vi "N Point Running Average.vi"(1 "n":i8, 2 "Input":dbl) -> (0 "Output":dbl)   [LabVIEW 2015]
uses:
  <vilib>/Analysis/baseanly.llb/Mean (DBL).vi
  <vilib>/Analysis/NI_AALBase.lvlib
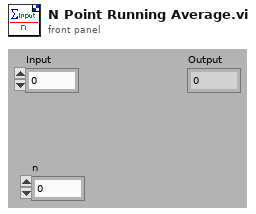
[diagram p1: front panel]
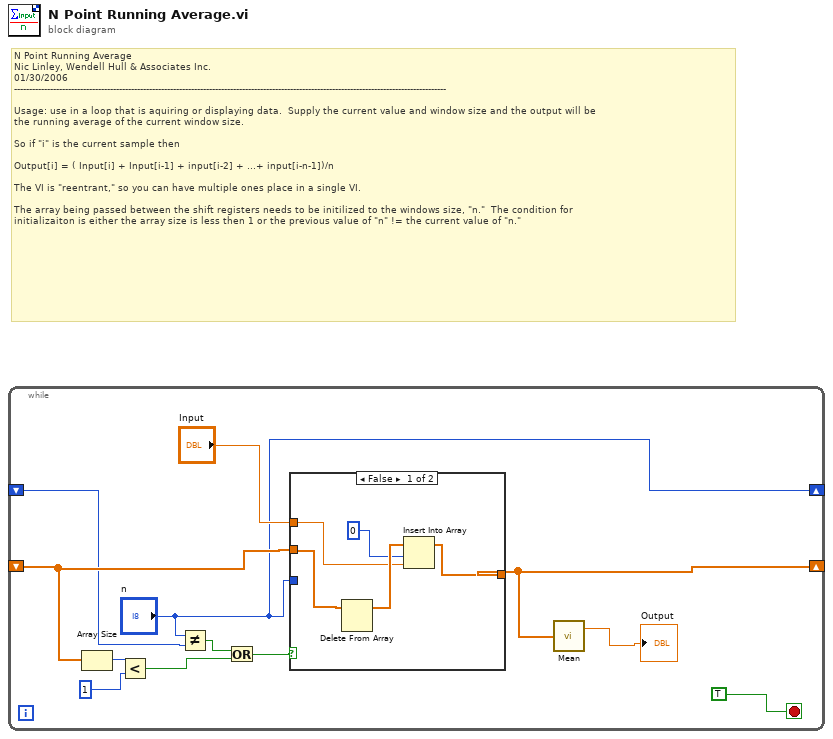
[diagram p0: block diagram]
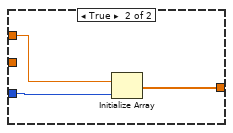
[diagram p2: hidden frame]
diagram:
  # "N Point Running Average \nNic Linley, Wendell Hull & Associates Inc.\n01/30/2006\n------------------------------------------------------------------------------------------------------------------------------------------------\n\nUsage: use in a loop that is aquiring or displaying data.  Supply the current value and window size and the output will be\nthe running average of the current window size.\n\nSo if \"i\" is the current sample then\n\nOutput[i] = ( Input[i] + Input[i-1] + input[i-2] + ...+ input[i-n-1])/n\n\nThe VI is \"reentrant,\" so you can have multiple ones place in a single VI.\n\nThe array being passed between the shift registers needs to be initilized to the windows size, \"n.\"  The condition for\ninitializaiton is either the array size is less then 1 or the previous value of \"n\" != the current value of \"n.\""
  n1 = while {
    shift-right: [w8] -> _
    shift-left: _ -> [w9]
    shift-right: ["n"] -> _
    shift-left: _ -> [w3]
    stop <- TRUE stop-if-true
    n2 = Array Size(array=w9) -> (size(s)=w11:i32)
    n3 = Less?(x=w11, y=1) -> (x < y?=w1:bool)
    n4 = Not Equal?(x="n", y=w3) -> (x != y?=w2:bool)
    n5 = Or(x=w2, y=w1) -> (x .or. y?=w5:bool)
    n6 = case shown="False" w5 {
      tunnel: "n" -> [_ w20]
      tunnel: "Input" -> [w15 w19]
      tunnel: [w14 w18] -> w8
      tunnel: w9 -> [w17 _]
      frame False {
        n7 = Delete From Array "Delete From Array"(array=w17) -> (array with subset deleted=w16:dbl[])  [unwired: 2 in, 1 out]
        n8 = Insert Into Array "Insert Into Array"(array=w16, index=0, new element=w15) -> (w14:dbl[])
      }
      frame True {
        n9 = Initialize Array "Initialize Array"(w19, w20) -> (w18:dbl[])
      }
    }
    n10 = call-poly <vilib>:"Mean.vi"("X"=w8) -> ("mean"=→"Output":dbl)  [unwired: 1 out]
  }
